vi "testZkAndDofIdx.vi"(8 "error in (no error)":errorcluster) -> (0 "error out":errorcluster)   [LabVIEW 2016]
doc: "Test the set/getZkAndDofInGroups.vi."
uses:
  ZTAAC/ZTAAC.lvclass
  StrictDef/InstName.ctl
  <vilib>/addons/_JKI Toolkits/Caraya/classes/Assert/Assert.lvclass
  <vilib>/addons/_JKI Toolkits/Caraya/classes/Test/Test.lvclass
  OfcFunc.lvlib
panel:
  in  "ZTAAC.lvclass":refnum<class "ZTAAC.lvclass">
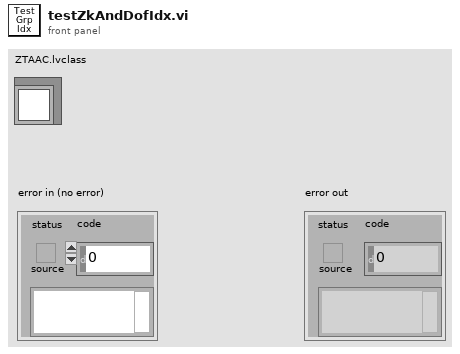
[diagram p1: front panel]
types:
  T1 = typedef "OfcFunc.lvlib/InstName.ctl" = enum16{"lsst", "comcam"}
  T2 = cluster{"Config Dir":path, "Inst Name":T1, "OptStateEsti Config File Name":string, "Mapping File Name":string, "Wavelength Table":string, "Intrinc Zk File Name":string, "y2 Corection File Name":string, "Index DOF File Name":string, "OptCtrl Config File Name":string, "State 0 File Name":string, "Weighting File Name":string, "PSSN Alpha File Name":string, "Authority Files":cluster{"Rigid Body Stroke File":string, "M1M3 Subsystem":cluster{"Mirror":string, "Actuatro Force File":string}, "M2 Subsystem":cluster{"Mirror":string, "Actuatro Force File":string}, "Num of Bending Mode":i32}, "Sensor Id to Name File Name":string, "Truncation Threshold":dbl, "Default Gain":dbl, "FWHM Threshold (arcsec)":dbl}
  T3 = cluster{"M2 Hexapod":bool[], "Cam Hexapod ":bool[], "M1M3 Bending Mode":bool[], "M2 Bending Mode":bool[]}
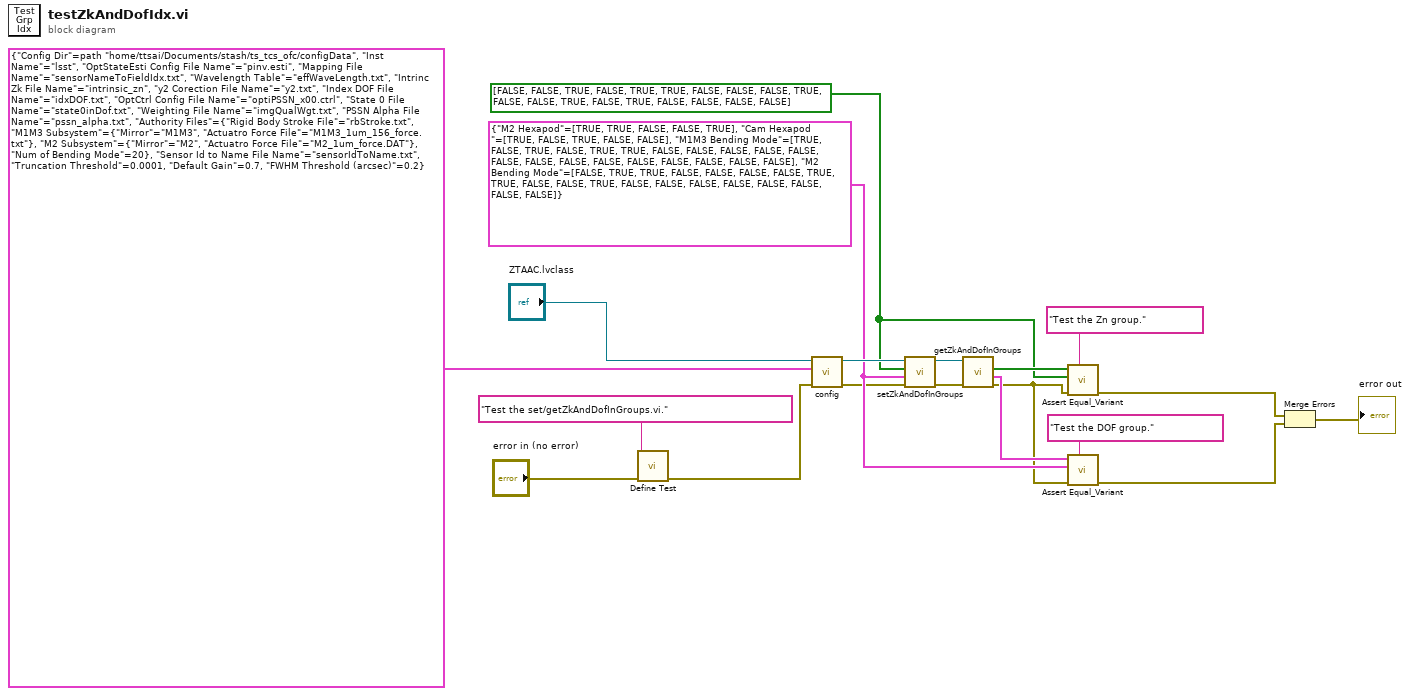
[diagram p0: block diagram]
diagram:
  w12 = T3 {"M2 Hexapod"=[TRUE, TRUE, FALSE, FALSE, TRUE], "Cam Hexapod "=[TRUE, FALSE, TRUE, FALSE, FALSE], "M1M3 Bending Mode"=[TRUE, FALSE, TRUE, FALSE, TRUE, TRUE, FALSE, FALSE, FALSE, FALSE, FALSE, FALSE, FALSE, FALSE, FALSE, FALSE, FALSE, FALSE, FALSE, FALSE], "M2 Bending Mode"=[FALSE, TRUE, TRUE, FALSE, FALSE, FALSE, FALSE, TRUE, TRUE, FALSE, FALSE, TRUE, FALSE, FALSE, FALSE, FALSE, FALSE, FALSE, FALSE, FALSE]} ("DOF in Groups")
  w15 = bool[] [FALSE, FALSE, TRUE, FALSE, TRUE, TRUE, FALSE, FALSE, FALSE, TRUE, FALSE, FALSE, TRUE, FALSE, TRUE, FALSE, FALSE, FALSE, FALSE] ("zn3Idx")
  n1 = call <vilib>:"Define Test.vi"("error in (no error)"="error in (no error)", "Label (VI Title)"="Test the set/getZkAndDofInGroups.vi.") -> ("error out"=w11:errorcluster)  [unwired: 9 in]
  n2 = call "config.vi"("error in (no error)"=w11, "ZTAAC Configuration"=T2 {"Config Dir"=path "/home/ttsai/Documents/stash/ts_tcs_ofc/configData", "Inst Name"=enum."lsst", "OptStateEsti Config File Name"="pinv.esti", "Mapping File Name"="sensorNameToFieldIdx.txt", "Wavelength Table"="effWaveLength.txt", "Intrinc Zk File Name"="intrinsic_zn", "y2 Corection File Name"="y2.txt", "Index DOF File Name"="idxDOF.txt", "OptCtrl Config File Name"="optiPSSN_x00.ctrl", "State 0 File Name"="state0inDof.txt", "Weighting File Name"="imgQualWgt.txt", "PSSN Alpha File Name"="pssn_alpha.txt", "Authority Files"={"Rigid Body Stroke File"="rbStroke.txt", "M1M3 Subsystem"={"Mirror"="M1M3", "Actuatro Force File"="M1M3_1um_156_force.txt"}, "M2 Subsystem"={"Mirror"="M2", "Actuatro Force File"="M2_1um_force.DAT"}, "Num of Bending Mode"=20}, "Sensor Id to Name File Name"="sensorIdToName.txt", "Truncation Threshold"=0.0001, "Default Gain"=0.7, "FWHM Threshold (arcsec)"=0.2}, "ZTAAC in"="ZTAAC.lvclass") -> ("error out"=w10:errorcluster, "ZTAAC out"=w19:refnum<class "ZTAAC.lvclass">)  [unwired: 7 in]
  n3 = call "setZkAndDofInGroups.vi"("error in (no error)"=w10, "DOF in Groups"=w12, "zn3Idx"=w15, "ZTAAC in"=w19) -> ("error out"=w9:errorcluster, "ZTAAC out"=w17:refnum<class "ZTAAC.lvclass">)  [unwired: 6 in]
  n4 = call "getZkAndDofInGroups.vi"("error in (no error)"=w9, "ZTAAC in"=w17) -> ("error out"=w8:errorcluster, "DOF in Groups"=w14:T3, "zn3Idx"=w16:bool[])  [unwired: 6 in, 1 out]
  n5 = call <vilib>:"Assert Equal_Variant.vi"("Label"="Test the Zn group.", "error in (no error)"=w8, "Y"=w15, "X"=w16) -> ("error out"=w7:errorcluster)  [unwired: 7 in]
  n6 = call <vilib>:"Assert Equal_Variant.vi"("Label"="Test the DOF group.", "error in (no error)"=w8, "Y"=w12, "X"=w14) -> ("error out"=w6:errorcluster)  [unwired: 7 in]
  n7 = Merge Errors(w7, w6) -> (→"error out":errorcluster)
